vi "MCL Wfma Trigger And Read.vi"(7 "handle":i32, 9 "wfAdcZ":dbl, 10 "wfAdcY":dbl, 11 "wfAdcX":dbl) -> (1 "wfAdcZ out":dbl, 2 "wfAdcY out":dbl, 3 "wfAdcX out":dbl, 5 "function return":i32)   [LabVIEW 2017, in "Madlib.lvlib"]
doc: "MADLIB_API int MCL_WfmaTriggerAndRead(double *wfAdcX, double *wfAdcY, double *wfAdcZ, int handle);"
uses:
  Madlib.lvlib
  Madlib.dll
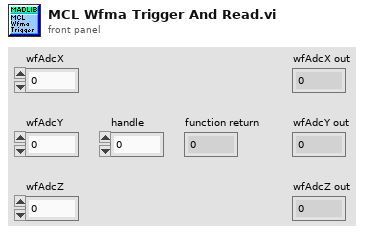
[diagram p1: front panel]
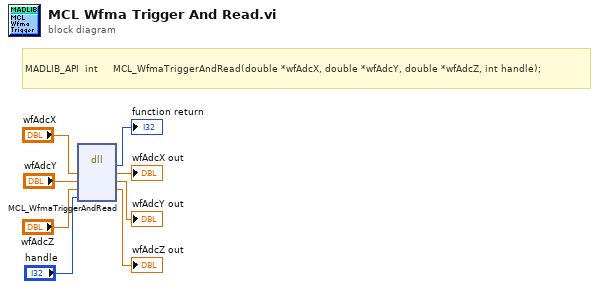
[diagram p0: block diagram]
diagram:
  # "MADLIB_API  int     MCL_WfmaTriggerAndRead(double *wfAdcX, double *wfAdcY, double *wfAdcZ, int handle);"
  n1 = dll-call lib="C:/Users/francesco/dev/pump-probe/Piezo/lvlib/Madlib.*" fn="MCL_WfmaTriggerAndRead"("wfAdcX"="wfAdcX", "wfAdcY"="wfAdcY", "wfAdcZ"="wfAdcZ", "handle"="handle") -> (→"function return":i32, "wfAdcX"=→"wfAdcX out":dbl, "wfAdcY"=→"wfAdcY out":dbl, "wfAdcZ"=→"wfAdcZ out":dbl)  [unwired: 4 in, 2 out]
